vi "Rd Wr settings Viewer Window Positions.vi"(7 "Window name":string, 8 "error in (no error)":errorcluster, 9 "Settings File":string="Viewer Windows.json", 10 "Write? (F:Read)":bool, 11 "Window Map":T3) -> (0 "error out":errorcluster, 1 "value":T1, 2 "Not Found?":bool, 3 "Window Map":T3)   [LabVIEW 2021]
uses:
  Chronos map Viewer Window List.ctl
  Chronos cluster Viewer Window.ctl
  <vilib>/Utility/miscctls.llb/LVRectTypeDef.ctl
  2e80df6d-94aa-46b9-8b94-ceea8c057880.vi
  659fb017-0e9f-42f9-b06e-930303f00cbc.vi
  <vilib>/JDP Science/JSONtext/Find Item.vi
  <vilib>/JDP Science/JSONtext/Next JSON Value.vi
  <vilib>/JDP Science/JSONtext/String Subset.vi
  <vilib>/JDP Science/JSONtext/Parsing/Advance past next JSON Value (inlined COPY).vi
  <vilib>/JDP Science/JSONtext/Parsing/Advance past whitespace.vi
  <vilib>/JDP Science/JSONtext/Parsing/Advance past String.vi
  <vilib>/JDP Science/JSONtext/Parsing/Advance past Number.vi
  <vilib>/JDP Science/JSONtext/Parsing/Advance past Line Ending.vi
  <vilib>/JDP Science/JSONtext/Parsing/Parse Full Path or Item Name.vi
  <vilib>/JDP Science/JSONtext/Parsing/Advance past Array.vi
  <vilib>/JDP Science/JSONtext/Parsing/Advance past Object.vi
  <vilib>/JDP Science/JSONtext/support/Error Cluster From Code.vi
  <vilib>/JDP Science/JSONtext/Offset/Find Item Locations by Path.vi
  <vilib>/JDP Science/JSONtext/JSON text to Variant.vi
  <vilib>/JDP Science/JSONtext/Variant to JSON Text.vi
  <vilib>/JDP Science/JSONtext/Set Item.vi
  <vilib>/JDP Science/JSONtext/LVClass Serializer/JSONtext LVClass Serializer.lvclass
panel:
  out "error out 2":errorcluster
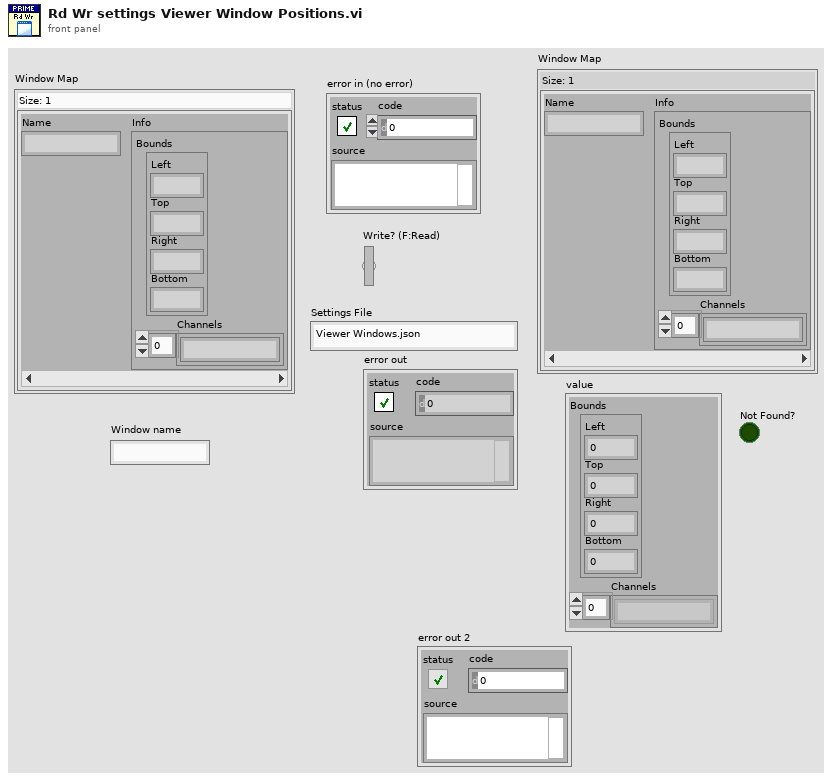
[diagram p1: front panel]
types:
  T1 = typedef "Chronos cluster Viewer Window.ctl" = cluster{"Bounds":T2, "Channels":string[]}
  T2 = typedef "LVRectTypeDef.ctl" = cluster{"Left":i16, "Top":i16, "Right":i16, "Bottom":i16}
  T3 = typedef "Chronos map Viewer Window List.ctl" = map{string, T1}
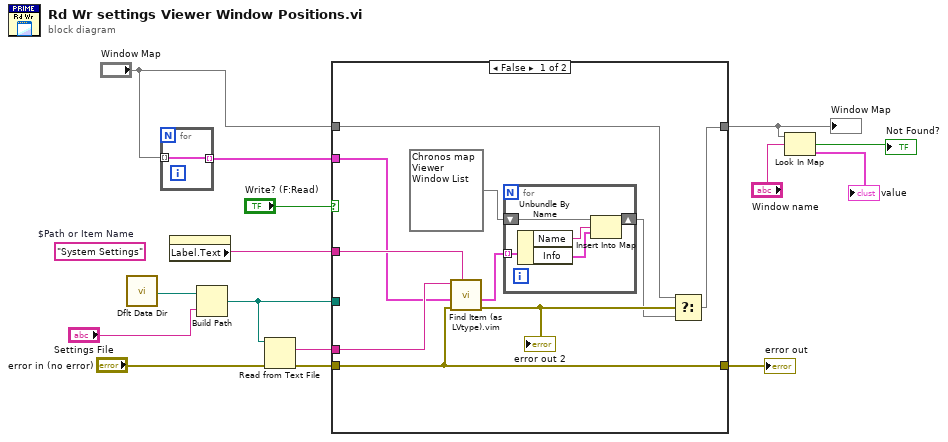
[diagram p0: block diagram]
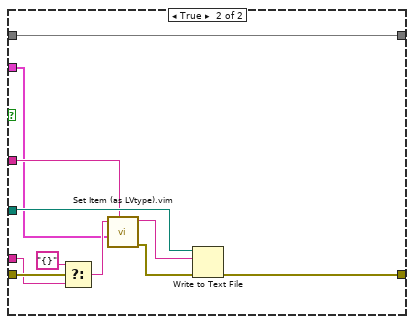
[diagram p2: hidden frame]
diagram:
  (unwired) "System Settings"  # $Path or Item Name
  n1 = call <vilib>:"Dflt Data Dir.vi"() -> ("App:Default Data Directory"=w13:path)
  n2 = for {
    tunnel: "Window Map" -> [w16] mode=indexing
    tunnel: [w16] -> w1 mode=indexing
  }
  n3 = property on="Map" class="Map (strict)"() -> ("Label.Text"=w7:string)  [unwired: 2 in, 2 out]
  n4 = Build Path(base path=w13, name or relative path="Settings File") -> (appended path=w8:path)
  n5 = Read from Text File(file (use dialog)=w8, error in="error in (no error)") -> (text=w9:string, error out=w10:errorcluster)  [unwired: 2 in, 2 out]
  n6 = case shown="False" "Write? (F:Read)" {
    tunnel: w10 -> [w22 w37]
    tunnel: "Window Map" -> [w21 w40]
    tunnel: w8 -> [_ w42]
    tunnel: [w22 w41] -> w12
    tunnel: [w26 w40] -> w6
    tunnel: w7 -> [w25 w39]
    tunnel: w9 -> [w23 w35]
    tunnel: w1 -> [w20 w32]
    frame False {
      n7 = call "Find Item (as LVtype).vim"("$Path or Item Name"=w25, "error in (no error)"=w22, "Data Type and Default Value"=w20, "JSON"=w23) -> ("error out"=w24:errorcluster, "Data"=w19:cluster{"Name":string, "Info":T1}[])  [unwired: 4 in, 2 out]
      "error out 2" <- w24
      n8 = for {
        tunnel: w19 -> [w29] mode=indexing
        shift-right: [w30] -> w17
        shift-left: T3 {} ("Window Map") -> [w31]
        n9 = Unbundle By Name(w29) -> ("Name"=w28:string, "Info"=w27:T1)
        n10 = Insert Into Map(map in=w31, key=w28, value=w27) -> (map out=w30:T3)  [unwired: 2 out]
      }
      n11 = Select(t=w21, s=w24, f=w17) -> (s? t:f=w26:T3)
    }
    frame True {
      n12 = Select(t="{}" ("JSON"), s=w37, f=w35) -> (s? t:f=w34:string)
      n13 = call "Set Item (as LVtype).vim"("$Path or Item Name"=w39, "Anything"=w32, "JSON"=w34) -> ("error out"=w33:errorcluster, "<JSON>"=w38:string)  [unwired: 5 in, 1 out]
      n14 = Write to Text File(file (use dialog)=w42, text=w38, error in=w33) -> (error out=w41:errorcluster)  [unwired: 1 in, 2 out]
    }
  }
  "error out" <- w12
  "Window Map" <- w6
  n15 = Look In Map(map=w6, key="Window name") -> (key not found?=→"Not Found?":bool, value=→"value":T1)  [unwired: 1 in]
